vi "Move the EXE.vi"(0 "Primary destination path":path, 11 "error in (no error)":errorcluster) -> (15 "error out":errorcluster)   [LabVIEW 2021, in "Packager Helpers.lvlib"]
uses:
  Packager Helpers.lvlib
  Path Functions/Path Functions.lvlib
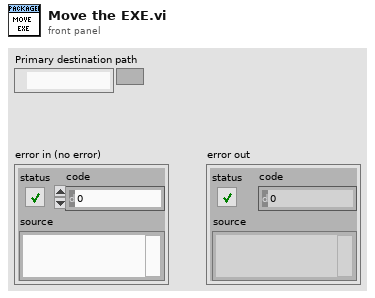
[diagram p1: front panel]
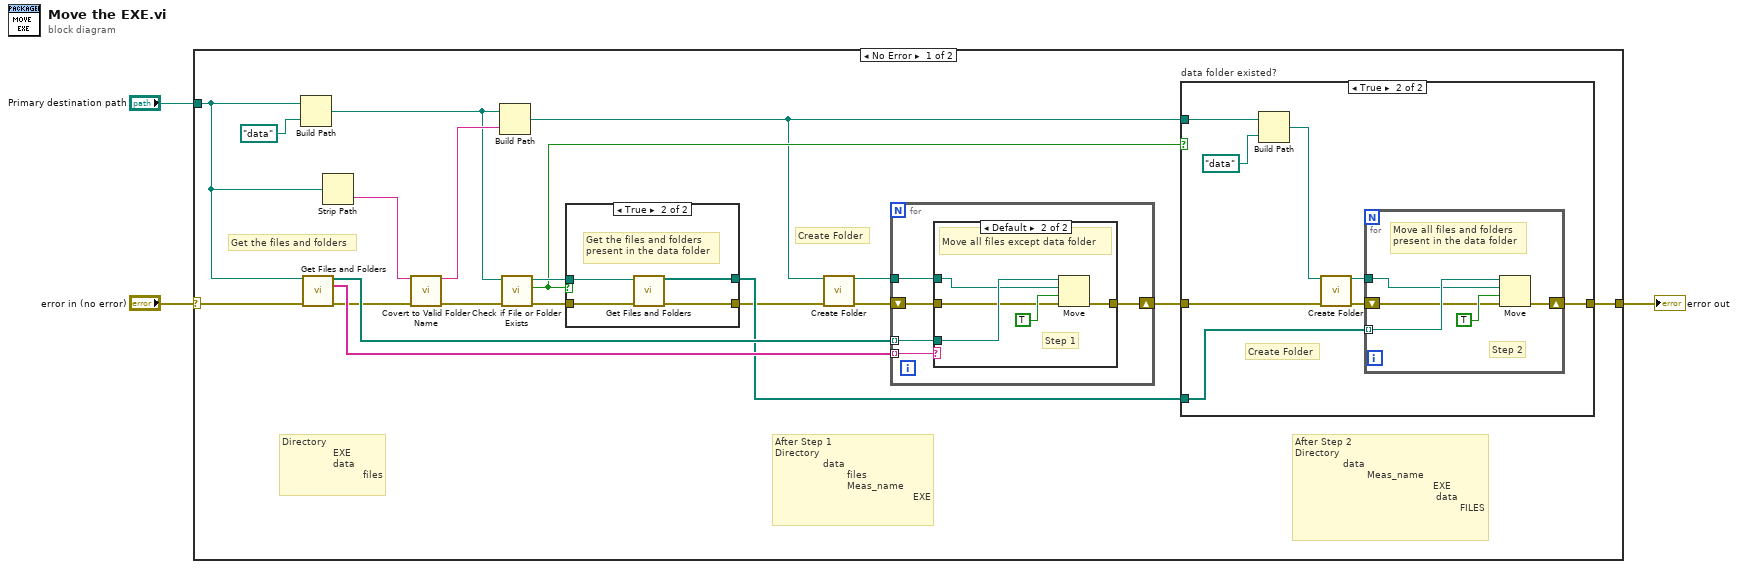
[diagram p0: block diagram]
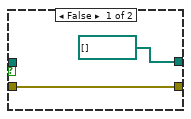
[diagram p3: hidden frame]
diagram:
  n1 = case shown="No Error" "error in (no error)" {
    selector: "error in (no error)" -> [w12 w55]
    tunnel: "Primary destination path" -> [w23 _]
    tunnel: [w4 w55] -> w1
    frame No Error {
      # "Directory\n                 EXE\n                 data\n                           files"
      # "Create Folder"
      # "Get the files and folders"
      # "After Step 2\nDirectory\n                data\n                        Meas_name\n                                              EXE\n                                               data\n                                                       FILES"
      # "After Step 1\nDirectory\n                data\n                        files\n                        Meas_name\n                                              EXE"
      n2 = Build Path(base path=w23, name or relative path=path "data") -> (appended path=w16:path)
      n3 = call "Get Files and Folders.vi"("File Directory"=w23, "error in (no error)"=w12) -> ("Files and Folders"=w20:path[], "Files and Folder Names"=w19:string[], "error out"=w11:errorcluster)  [unwired: 11 in]
      n4 = Strip Path(path=w23) -> (name=w22:string)  [unwired: 1 out]
      n5 = call "Covert to Valid Folder Name.vi"("Folder Name"=w22, "error in (no error)"=w11) -> ("Valid Folder Name"=w21:string, "error out"=w10:errorcluster)  [unwired: 12 in]
      n6 = Build Path(base path=w16, name or relative path=w21) -> (appended path=w5:path)
      n7 = call <vilib>:"Check if File or Folder Exists.vi"("error in (no error)"=w10, "path"=w16) -> ("error out"=w9:errorcluster, "file or folder exists?"=w14:bool, "dup path"=w15:path)  [unwired: 7 in]
      n8 = case shown="True" w14 {
        tunnel: w9 -> [w35 w38]
        tunnel: [w35 w37] -> w8
        tunnel: [path[] [] ("Files and Folders") w40] -> w17
        tunnel: w15 -> [_ w39]
        frame False {
        }
        frame True {
          # "Get the files and folders\npresent in the data folder"
          n9 = call "Get Files and Folders.vi"("File Directory"=w39, "error in (no error)"=w38) -> ("Files and Folders"=w40:path[], "error out"=w37:errorcluster)  [unwired: 11 in, 1 out]
        }
      }
      n10 = call "Create Folder.vi"("Directory Path"=w5, "error in (no error)"=w8) -> ("Dup Directory Path"=w13:path, "error out"=w7:errorcluster)  [unwired: 12 in]
      n11 = for {
        tunnel: w20 -> [w27] mode=indexing
        shift-right: [w24] -> w18
        shift-left: w7 -> [w25]
        tunnel: w19 -> [w28] mode=indexing
        tunnel: w13 -> [w26]
        n12 = case shown="Default" w28 {
          tunnel: w27 -> [_ w34]
          tunnel: w25 -> [w29 w31]
          tunnel: w26 -> [_ w32]
          tunnel: [w29 w30] -> w24
          frame "data" {
          }
          frame Default {
            # "Step 1"
            # "Move all files except data folder"
            n13 = Move(source path=w34, error in=w31, 9:TRUE ("overwrite (F)"), 10:w32) -> (error out=w30:errorcluster)  [unwired: 1 in, 2 out]
          }
        }
      }
      n14 = case "data folder existed?" shown="True" w14 {
        tunnel: w18 -> [w41 w46]
        tunnel: w17 -> [_ w47]
        tunnel: [w41 w44] -> w4
        tunnel: w5 -> [_ w42]
        frame False {
        }
        frame True {
          # "Create Folder"
          n15 = Build Path(base path=w42, name or relative path=path "data") -> (appended path=w49:path)
          n16 = call "Create Folder.vi"("Directory Path"=w49, "error in (no error)"=w46) -> ("Dup Directory Path"=w48:path, "error out"=w45:errorcluster)  [unwired: 12 in]
          n17 = for {
            tunnel: w47 -> [w54] mode=indexing
            tunnel: w48 -> [w53]
            shift-right: [w50] -> w44
            shift-left: w45 -> [w51]
            # "Move all files and folders\npresent in the data folder"
            # "Step 2"
            n18 = Move(source path=w54, error in=w51, 9:TRUE ("overwrite (F)"), 10:w53) -> (error out=w50:errorcluster)  [unwired: 1 in, 2 out]
          }
        }
      }
    }
    frame Error {
    }
  }
  "error out" <- w1
